vi "8_Direct_Time_Tag_Stream_Access.vi"() -> ()   [LabVIEW 2015]
uses:
  C:/Users/MX-Microscope/Documents/LabVIEW Data/lvoop_campus_2018/Detector_Class/Swabian/time_tagger_vis/TTCSharp32.dll
  TTCSharp32.dll
panel:
  out "size(s)":i32
  out "number of time tags 2":i32
  out "hasOverflows 2":bool
  out "sumChannel 2":u32
  out "sumTime 2":i64
  out "tagTimestamps 2":i64[](array[numeric])
  out "tagChannels 2":u32[](array[numeric])
  out "tagChannels":u32[](array[numeric])
  out "tagTimestamps":i64[](array[numeric])
  out "sumTime":i64
  out "sumChannel":u32
  out "hasOverflows":bool
  in  "Data rate":dbl=8.0
  out "loop iteration":i32
  out "number of time tags":i32
  # "x 0.9 Million samples / s"
  # "We aquire the data of the raw time tag stream 1000 times\nevery 1s."
  # "The number of time tags received should not increase\npermantently otherwise the average data rate is too high \nand the cpu cannot handle the time tag stream which of \ncourse depends highly on the evaluation performed."
  # "Evaluation"
  # "The evaluation done here is useless - but out of each tag the time and channel information\nis used to calculate something. The evaluation method will limit the number of tags which can be used.\n\nFor a i7-5600U the full maximum transfer rate limited by the USB bandwidth (~8-9 million tags per second) can be evaluated"
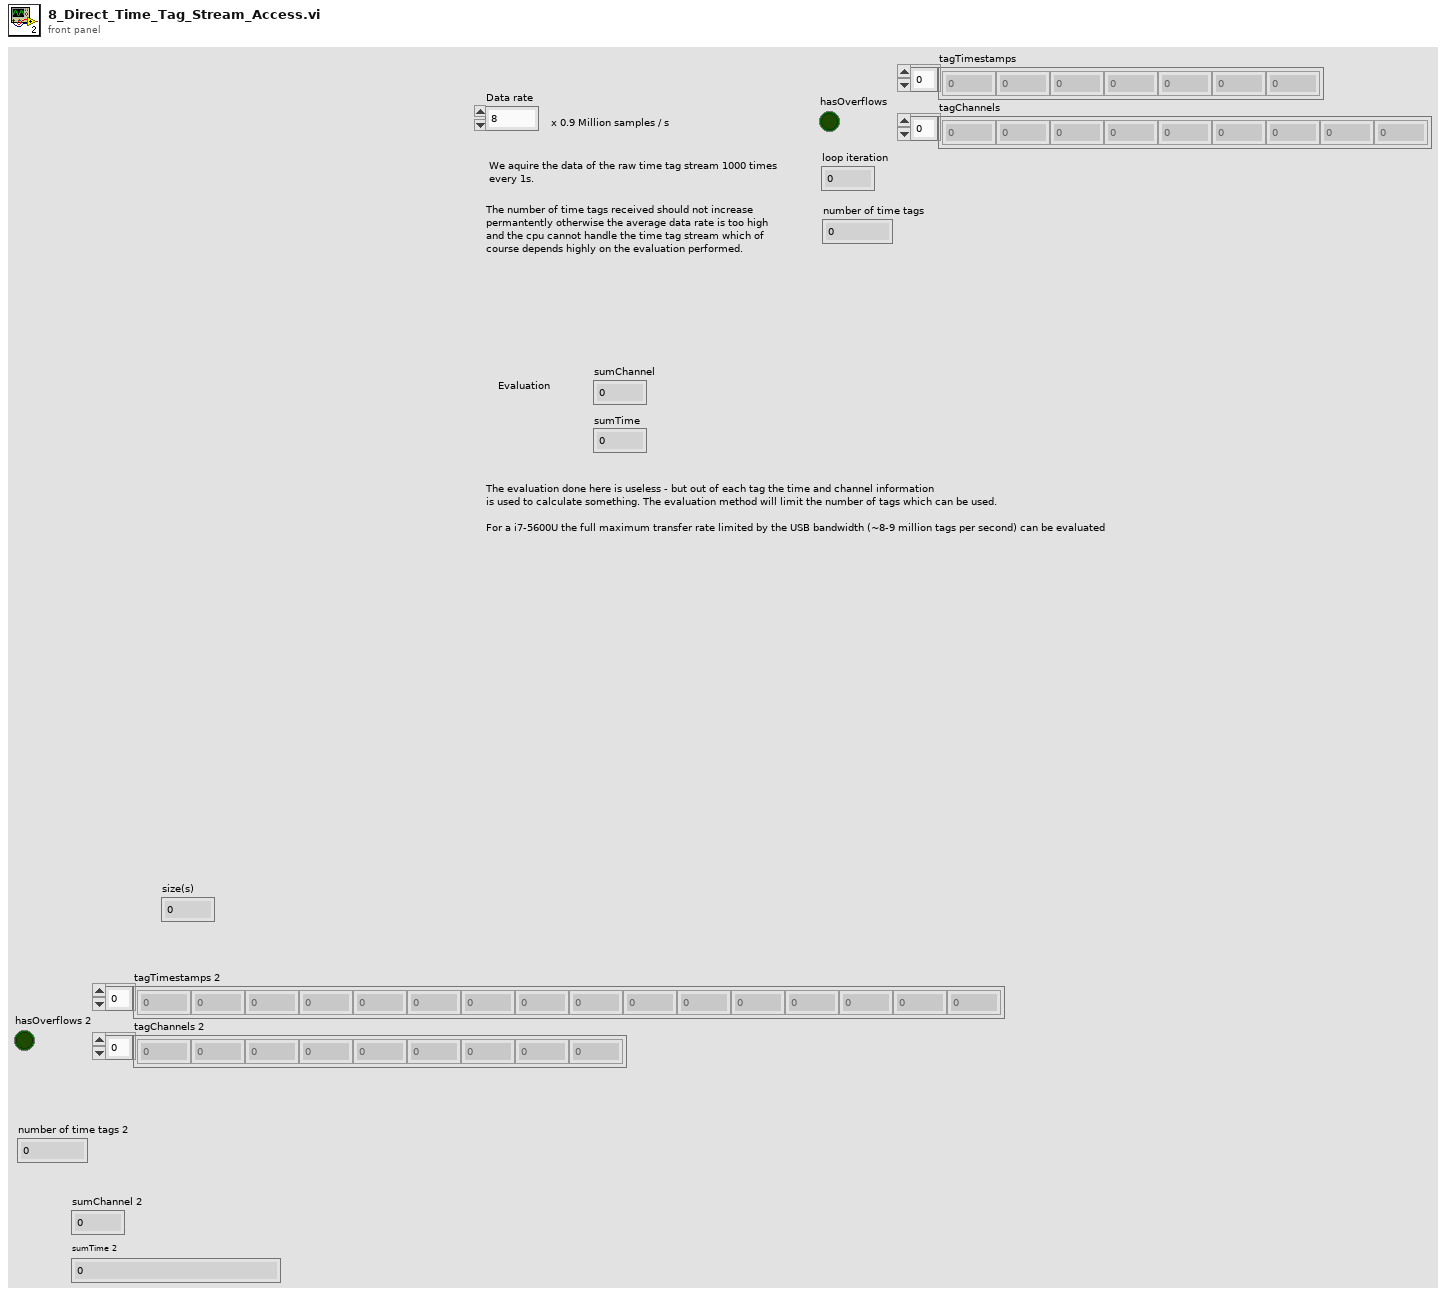
[diagram p1: front panel]
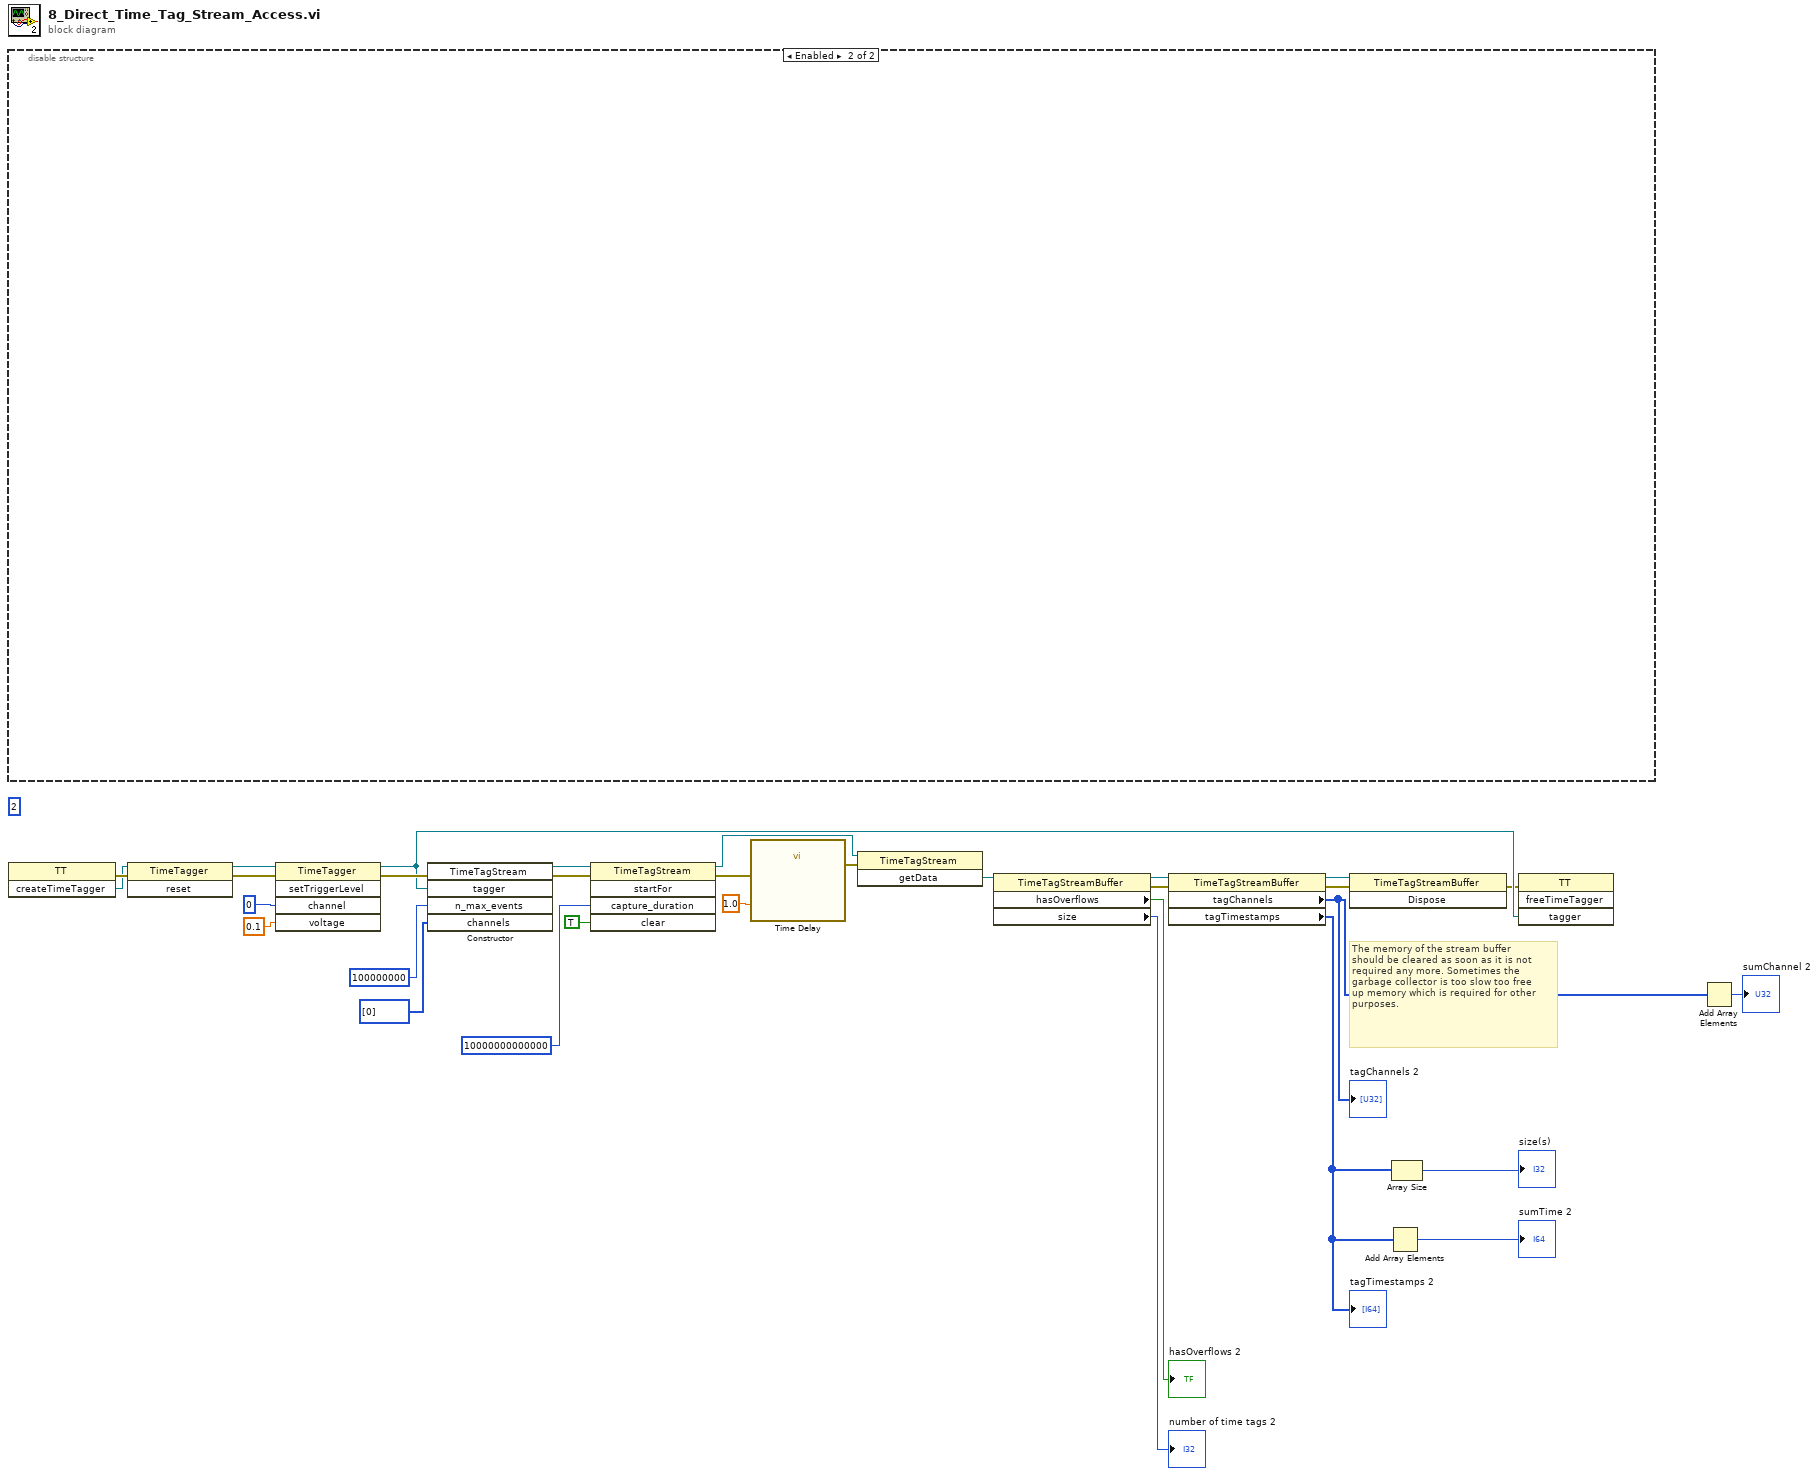
[diagram p0: block diagram]
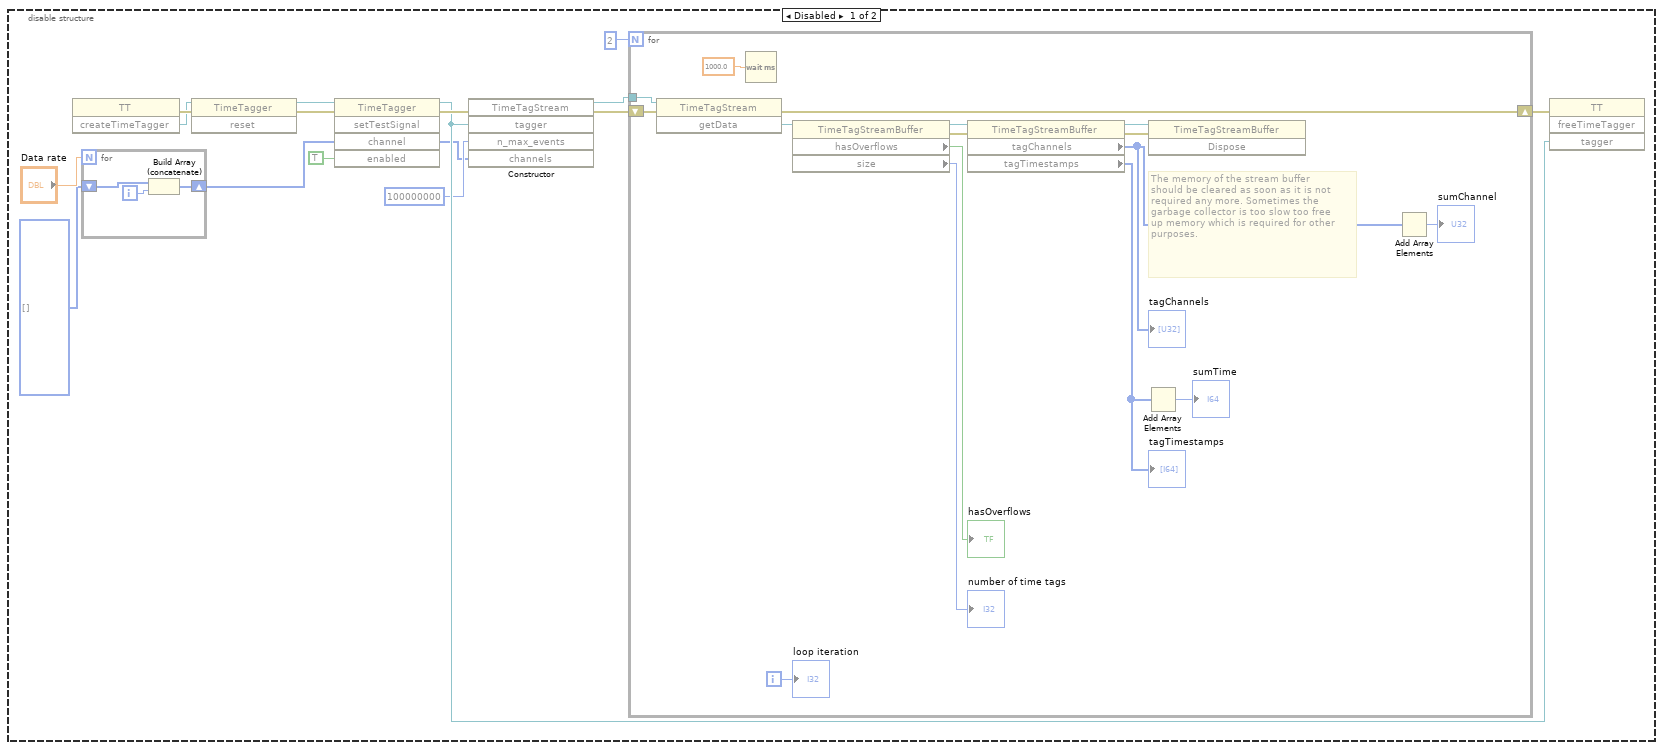
[diagram p2: hidden frame]
diagram:
  (unwired) 2
  # "The memory of the stream buffer \nshould be cleared as soon as it is not\nrequired any more. Sometimes the\ngarbage collector is too slow too free\nup memory which is required for other\npurposes."
  n1 = disable-structure shown="Enabled" {
    frame Disabled {
      n2 = invoke class="TT" method="createTimeTagger"() -> (error out=w47:errorcluster, "createTimeTagger"=w46:refnum<k24>)  [unwired: 3 in, 1 out]
      n3 = for {
        N: "Data rate" -> [_]
        shift-right: [w49] -> w36
        shift-left: i32[] [] -> [w48]
        i -> [w50]
        n4 = Build Array (concatenate)(w48, w50) -> (w49:i32[])
      }
      n5 = invoke class="TimeTagger" method="reset"(reference=w46, error in=w47) -> (reference out=w39:refnum<k24>, error out=w38:errorcluster)  [unwired: 1 in, 1 out]
      n6 = invoke class="TimeTagger" method="setTestSignal"(reference=w39, error in=w38, "channel"=w36, "enabled"=TRUE) -> (reference out=w34:refnum<k24>, error out=w37:errorcluster, "channel"=w32:u32[])  [unwired: 1 in, 2 out]
      n7 = constructor class="TimeTagStream"(error in=w37, "tagger"=w34, "n_max_events"=100000000, "channels"=w32) -> (reference out=w45:refnum<k24>, error out=w35:errorcluster)  [unwired: 2 in, 4 out]
      n8 = for {
        N: 2 -> [_]
        tunnel: w45 -> [w66]
        shift-right: [w65] -> w44
        shift-left: w35 -> [w61]
        i -> [w63]
        # "The memory of the stream buffer \nshould be cleared as soon as it is not\nrequired any more. Sometimes the\ngarbage collector is too slow too free\nup memory which is required for other\npurposes."
        n9 = invoke class="TimeTagStream" method="getData"(reference=w66, error in=w61) -> (error out=w65:errorcluster, "getData"=w64:refnum<k24>)  [unwired: 1 in, 1 out]
        n10 = Wait (ms)(milliseconds to wait=1000.0 ("Delay Time (s)")) -> ()  [unwired: 1 out]
        n11 = property class="TimeTagStreamBuffer"(reference=w64) -> (reference out=w57:refnum<k24>, error out=w58:errorcluster, "hasOverflows"=→"hasOverflows":bool, "size"=→"number of time tags":i32)  [unwired: 1 in]
        n12 = property class="TimeTagStreamBuffer"(reference=w57, error in=w58) -> (reference out=w51:refnum<k24>, error out=w52:errorcluster, "tagChannels"=w56:u32[], "tagTimestamps"=w55:i64[])
        "tagTimestamps" <- w55
        "tagChannels" <- w56
        n13 = Add Array Elements(numeric array=w55) -> (sum=→"sumTime":i64)
        n14 = invoke class="TimeTagStreamBuffer" method="Dispose"(reference=w51, error in=w52) -> ()  [unwired: 1 in, 3 out]
        n15 = Add Array Elements(numeric array=w56) -> (sum=→"sumChannel":u32)
        "loop iteration" <- w63
      }
      n16 = invoke class="TT" method="freeTimeTagger"(error in=w44, "tagger"=w34) -> ()  [unwired: 2 in, 4 out]
    }
    frame Enabled {
    }
  }
  n17 = invoke class="TT" method="createTimeTagger"() -> (error out=w31:errorcluster, "createTimeTagger"=w30:refnum<k24>)  [unwired: 3 in, 1 out]
  n18 = invoke class="TimeTagger" method="reset"(reference=w30, error in=w31) -> (reference out=w25:refnum<k24>, error out=w27:errorcluster)  [unwired: 1 in, 1 out]
  n19 = invoke class="TimeTagger" method="setTriggerLevel"(reference=w25, error in=w27, "channel"=u32 0, "voltage"=0.1) -> (reference out=w24:refnum<k24>, error out=w26:errorcluster)  [unwired: 1 in, 3 out]
  n20 = constructor class="TimeTagStream"(error in=w26, "tagger"=w24, "n_max_events"=100000000, "channels"=u32[] [0]) -> (reference out=w20:refnum<k24>, error out=w21:errorcluster)  [unwired: 2 in, 4 out]
  n21 = invoke class="TimeTagStream" method="startFor"(reference=w20, error in=w21, "capture_duration"=i64 10000000000000, "clear"=TRUE) -> (reference out=w19:refnum<k24>, error out=w3:errorcluster)  [unwired: 1 in, 3 out]
  n22 = call "Time Delay"("error in (no error)"=w3, "Delay Time (s)"=1.0) -> ("error out"=w2:errorcluster)  [unwired: 9 in]
  n23 = invoke class="TimeTagStream" method="getData"(reference=w19, error in=w2) -> ("getData"=w18:refnum<k24>)  [unwired: 1 in, 2 out]
  n24 = property class="TimeTagStreamBuffer"(reference=w18) -> (reference out=w14:refnum<k24>, error out=w15:errorcluster, "hasOverflows"=→"hasOverflows 2":bool, "size"=→"number of time tags 2":i32)  [unwired: 1 in]
  n25 = property class="TimeTagStreamBuffer"(reference=w14, error in=w15) -> (reference out=w9:refnum<k24>, error out=w10:errorcluster, "tagChannels"=w13:u32[], "tagTimestamps"=w8:i64[])
  "tagTimestamps 2" <- w8
  "tagChannels 2" <- w13
  n26 = invoke class="TimeTagStreamBuffer" method="Dispose"(reference=w9, error in=w10) -> (error out=w4:errorcluster)  [unwired: 1 in, 2 out]
  n27 = Add Array Elements(numeric array=w8) -> (sum=→"sumTime 2":i64)
  n28 = Array Size(array=w8) -> (size(s)=→"size(s)":i32)
  n29 = invoke class="TT" method="freeTimeTagger"(error in=w4, "tagger"=w24) -> ()  [unwired: 2 in, 4 out]
  n30 = Add Array Elements(numeric array=w13) -> (sum=→"sumChannel 2":u32)
